vi "WaitBallOrientSkill.vi"(6 "Role ofRobotThat\nmake the pass":T1=enum."PassKicker", 8 "error in (no error)":errorcluster, 9 "Robot":refnum<class "Robot.lvclass">, 10 "Game":refnum<class "Game.lvclass">, 11 "WaitBallOrientSkill in":refnum<class "WaitBallOrientSkill.lvclass">) -> (0 "error out":errorcluster, 2 "robot out":refnum<class "Robot.lvclass">, 3 "WaitBallOrientSkill out":refnum<class "WaitBallOrientSkill.lvclass">)   [LabVIEW 2023, in "WaitBallOrientSkill.lvclass"]
uses:
  WaitBallOrientSkill.lvclass
  Robot_class/Robot.lvclass
  Game_class/Game.lvclass
  Robot_class/roles.ctl
  Object_class/Object.lvclass/Object.ctl
  Game_class/Game.lvclass/Game.ctl
  Team_class/Team.lvclass/Team.ctl
  Robot_class/Robot.lvclass/Robot.ctl
  Game_class/Read BallRef.vi
  Game_class/Read Utilities.lvclass.vi
  Game_class/Read FieldRef.vi
  Game_class/Read OffensiveTeam.vi
  Team_class/Read RobotRef.vi
  Object_class/Read x.vi
  Object_class/Read y.vi
  Robot_class/Read orientation.vi
  Robot_class/Write dest_x.vi
  Robot_class/Write dest_y.vi
  Robot_class/Write dest_orientation.vi
  Ally_class/Ally.lvclass
  Ball_class/Ball.lvclass
  Utilities_class/Utilities.lvclass
  Field_class/Field.lvclass
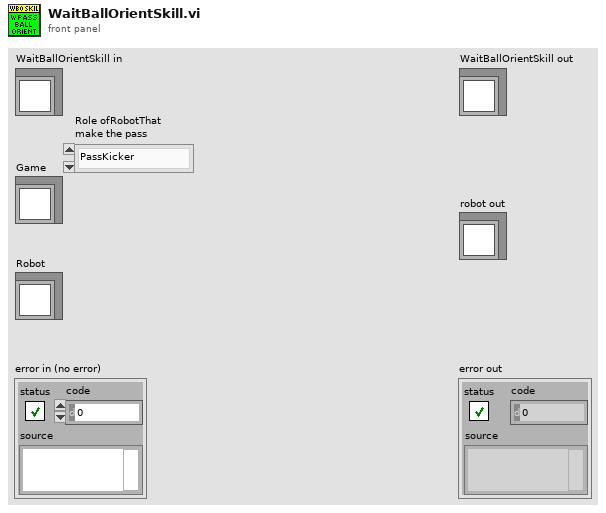
[diagram p1: front panel]
types:
  T1 = typedef "roles.ctl" = enum16{"BallChallengerAttackerVSS", "NormalAttackerVSS", "AttackerAimGoalVSS", "DefenderAreaVSS", "KeeperVSS", "Tabler", "TableFinalizer", "PrepareRollToPassRoller", "PrepareRollToPassReceiver", "SimplePassRoll", "SimplePassRollReceiver", "PenaltyDefense", "PreparePassReceiver 2", "PreparePassReceiver 1", "PassObserver", "Timeout", "Goto", "ZigZag", "None", "BallOutOfField", "DefenderArea", "Duelist", "AttackerStop", "FollowAttacker", "KeeperRole", "KickPenalty", "AttackerAimGoal", "AttackerBlock", "Marker", "Halt", "Shoot", "PassKicker", "PassReceiver", "TestRole", "PenaltyAttacker"}
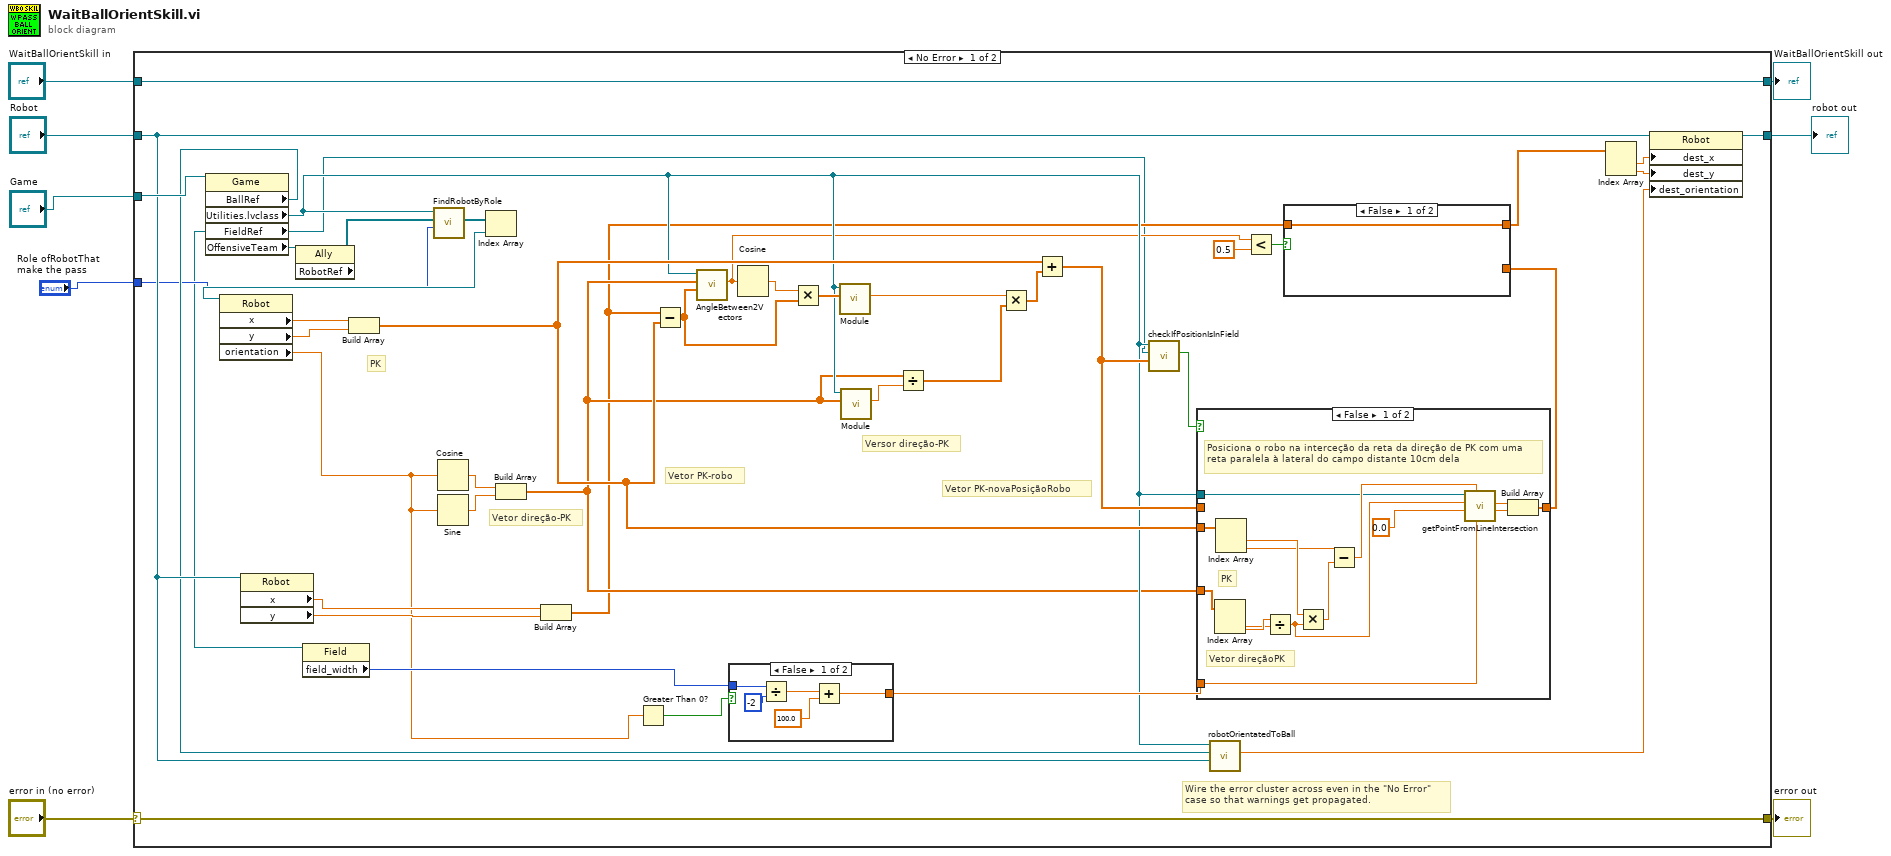
[diagram p0: block diagram]
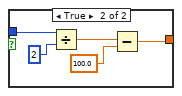
[diagram p4: hidden frame]
diagram:
  n1 = case shown="No Error" "error in (no error)" {
    selector: "error in (no error)" -> [w50 w81]
    tunnel: [w50 w81] -> w7
    tunnel: [w51 w80] -> w5
    tunnel: "WaitBallOrientSkill in" -> [w51 w80]
    tunnel: "Robot" -> [w26 _]
    tunnel: [w32 _] -> w3
    tunnel: "Game" -> [w27 _]
    tunnel: "Role ofRobotThat\nmake the pass" -> [w11 _]
    frame No Error {
      # "Versor direção-PK"
      # "PK"
      # "Vetor direção-PK"
      # "Vetor PK-novaPosiçãoRobo"
      # "Vetor PK-robo"
      # "Wire the error cluster across even in the \"No Error\"\ncase so that warnings get propagated."
      n2 = property class="Game"(reference=w27) -> ("BallRef"=w12:refnum<class "Ball.lvclass">, "Utilities.lvclass"=w21:refnum<class "Utilities.lvclass">, "FieldRef"=w9:refnum<class "Field.lvclass">, "OffensiveTeam"=w38:refnum<class "Ally.lvclass">)  [unwired: 1 in, 2 out]
      n3 = property class="Robot"(reference=w26) -> ("x"=w49:dbl, "y"=w48:dbl)  [unwired: 1 in, 2 out]
      n4 = property class="Ally"(reference=w38) -> ("RobotRef"=w37:refnum<class "Robot.lvclass">[])  [unwired: 1 in, 2 out]
      n5 = property class="Field"(reference=w9) -> ("field_width"=w42:i32)  [unwired: 1 in, 2 out]
      n6 = call "FindRobotByRole.vi"("role"=w11, "RobotRef"=w37, "Utilities in"=w21) -> ("Robots"=w35:refnum<class "Robot.lvclass">[])  [unwired: 6 in, 2 out]
      n7 = Index Array(array=w35) -> (element=w36:refnum<class "Robot.lvclass">)  [unwired: 1 in]
      n8 = property class="Robot"(reference=w36) -> ("x"=w34:dbl, "y"=w33:dbl, "orientation"=w28:dbl)  [unwired: 1 in, 2 out]
      n9 = Build Array(w34, w33) -> (w29:dbl[])
      n10 = Cosine(x=w28) -> (cos(x)=w31:dbl)
      n11 = Sine(x=w28) -> (sin(x)=w30:dbl)
      n12 = Build Array(w31, w30) -> (w19:dbl[])
      n13 = Build Array(w49, w48) -> (w15:dbl[])
      n14 = Greater Than 0?(x=w28) -> (x > 0?=w43:bool)
      n15 = Subtract(x=w15, y=w29) -> (x-y=w47:dbl[])
      n16 = call "AngleBetween2Vectors.vi"("Array 1"=w47, "Array 2"=w19, "Utilities in"=w21) -> ("Numeric"=w16:dbl)  [unwired: 6 in, 2 out]
      n17 = case shown="False" w43 {
        tunnel: w42 -> [w73 w79]
        tunnel: [w72 w77] -> w41
        frame False {
          n18 = Divide(x=w73, y=-2) -> (x/y=w71:dbl)
          n19 = Add(x=w71, y=100.0) -> (x+y=w72:dbl)
        }
        frame True {
          n20 = Divide(x=w79, y=2) -> (x/y=w76:dbl)
          n21 = Subtract(x=w76, y=100.0) -> (x-y=w77:dbl)
        }
      }
      n22 = Cosine(x=w16) -> (cos(x)=w46:dbl)
      n23 = Multiply(x=w46, y=w47) -> (x*y=w24:dbl[])
      n24 = call-dynamic "Module.vi"("2D vector"=w24, "Utilities in"=w21) -> ("Modulo"=w22:dbl)  [unwired: 7 in, 2 out]
      n25 = call-dynamic "Module.vi"("2D vector"=w19, "Utilities in"=w21) -> ("Modulo"=w18:dbl)  [unwired: 7 in, 2 out]
      n26 = Divide(x=w19, y=w18) -> (x/y=w20:dbl[])
      n27 = Multiply(x=w22, y=w20) -> (x*y=w23:dbl[])
      n28 = Add(x=w29, y=w23) -> (x+y=w44:dbl[])
      n29 = call "checkIfPositionIsInField.vi"("Position"=w44, "FieldRef"=w9, "Utilities in"=w21) -> ("Position Is In Field?"=w45:bool)  [unwired: 4 in, 4 out]
      n30 = case shown="False" w45 {
        tunnel: w44 -> [_ w69]
        tunnel: [w66 w69] -> w13
        tunnel: w41 -> [w64 _]
        tunnel: w29 -> [w63 _]
        tunnel: w19 -> [w62 _]
        tunnel: w21 -> [w54 _]
        frame False {
          # "PK"
          # "Vetor direçãoPK"
          # "Posiciona o robo na interceção da reta da direção de PK com uma reta paralela à lateral do campo distante 10cm dela"
          n31 = Index Array(array=w62) -> (element #1=w60:dbl, element #2=w61:dbl)  [unwired: 2 in]
          n32 = Index Array(array=w63) -> (element #1=w59:dbl, element #2=w58:dbl)  [unwired: 2 in]
          n33 = Divide(x=w61, y=w60) -> (x/y=w55:dbl)
          n34 = Multiply(x=w59, y=w55) -> (x*y=w57:dbl)
          n35 = Subtract(x=w58, y=w57) -> (x-y=w56:dbl)
          n36 = call "getPointFromLineIntersection.vi"("b2"=w64, "b1"=w56, "a2"=0.0, "a1"=w55, "Utilities in"=w54) -> ("y_intersection"=w67:dbl, "x_intersection"=w68:dbl)  [unwired: 3 in, 2 out]
          n37 = Build Array(w68, w67) -> (w66:dbl[])
        }
        frame True {
        }
      }
      n38 = call "robotOrientatedToBall.vi"("Robot"=w26, "BallRef"=w12, "Utilities in"=w21) -> ("Orientation"=w25:dbl)  [unwired: 6 in, 2 out]
      n39 = Less?(x=w16, y=0.5) -> (x < y?=w10:bool)
      n40 = case shown="False" w10 {
        tunnel: w15 -> [w52 _]
        tunnel: [w52 w53] -> w14
        tunnel: w13 -> [_ w53]
        frame False {
        }
        frame True {
        }
      }
      n41 = Index Array(array=w14) -> (element #1=w40:dbl, element #2=w39:dbl)  [unwired: 2 in]
      n42 = property class="Robot"(reference=w26, "dest_x"=w40, "dest_y"=w39, "dest_orientation"=w25) -> (reference out=w32:refnum<class "Robot.lvclass">)  [unwired: 1 in, 1 out]
    }
    frame Error {
    }
  }
  "error out" <- w7
  "WaitBallOrientSkill out" <- w5
  "robot out" <- w3
